vi "jitter.vi"(6 "delta":dbl, 11 "in":dbl) -> (3 "out":dbl)   [LabVIEW 2019]
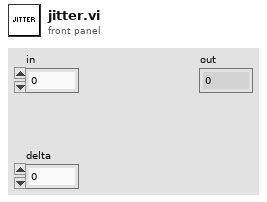
[diagram p1: front panel]
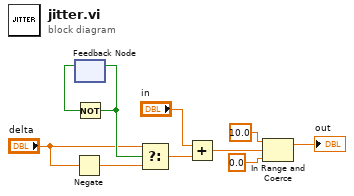
[diagram p0: block diagram]
diagram:
  n1 = Negate(x="delta") -> (-x=w7:dbl)
  n2 = feedback #1() -> (w10:bool)  [unwired: 1 in]
  n3 = Not(x=w10) -> (.not. x?=w9:bool)
  n4 = feedback-in #1(w9) -> ()
  n5 = Select(t="delta", s=w9, f=w7) -> (s? t:f=w6:dbl)
  n6 = Add(x="in", y=w6) -> (x+y=w2:dbl)
  n7 = In Range and Coerce(upper limit=10.0, x=w2, lower limit=0.0) -> (coerced(x)=→"out":dbl)  [unwired: 1 out]
